vi "Pattern  Gen Test.vi"() -> ()   [LabVIEW 2016]
uses:
  Classes/Config_Read/Config_Read.lvclass
  Classes/BML_Frame_SetID/BML_Frame_SetID.lvclass
  C:/Users/Zijun/Desktop/zijun_PXI_dev/Solutions/5g_eap/trunk/1.0/HiSi5GmmWave/BML_Pattern_Gen_Refactor/Classes/BML_Frame_Root/BML_Frame_Root.lvclass
  Classes/Config_Read/Frame_Data.ctl
  Classes/Config_Read/OperationMode.ctl
  Classes/Config_Read/BurstLength.ctl
  Classes/Config_Read/RW_Option.ctl
  Classes/BML_DigiPattern_Generator/BML_DigiPattern_Generator.lvclass
  Classes/BML_Frame_Write/BML_Frame_Write.lvclass
  Classes/BML_Frame_RW/BML_Frame_RW.lvclass
panel:
  out "error out":errorcluster
  in  "PinMap":path
  in  "ChipID":u8
  in  "Config Path":path
  in  "error in (no error)":errorcluster
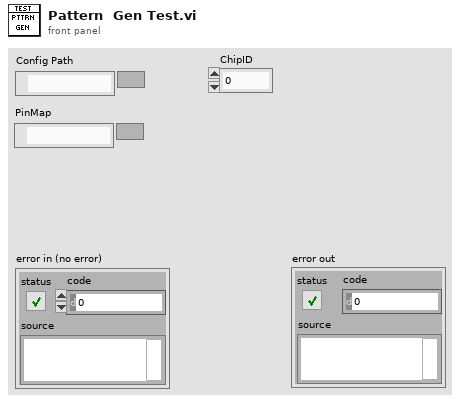
[diagram p1: front panel]
types:
  T1 = typedef "Config_Read.lvclass/Frame_Data.ctl" = cluster{"Pattern_Name":string, "Operation Mode":T2, "BurstLength":T3, "FSN":u8, "Start_Addr":u16, "Data":u8[], "R/W?":T4}
  T2 = typedef "Config_Read.lvclass/OperationMode.ctl" = enum8{"Normal", "ImmeEffect", "InitSlaveID", "LoadData"}
  T3 = typedef "Config_Read.lvclass/BurstLength.ctl" = enum8{"0", "2", "3", "4", "5", "8", "16", "32"}
  T4 = typedef "Config_Read.lvclass/RW_Option.ctl" = enum16{"Read", "Write", "R/W"}
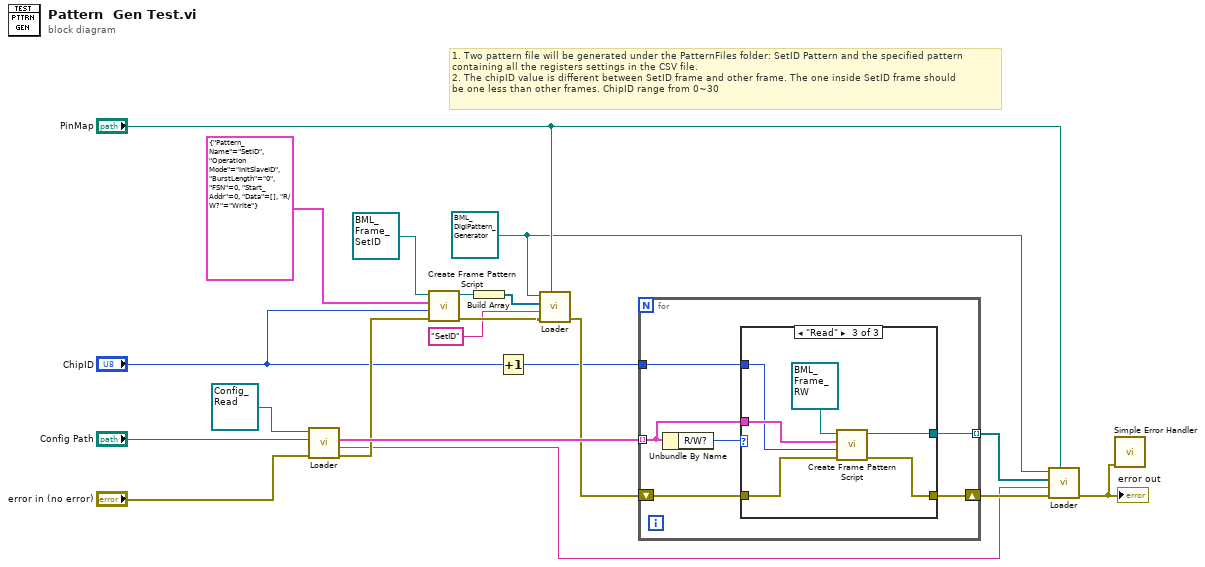
[diagram p0: block diagram]
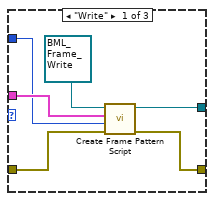
[diagram p2: hidden frame]
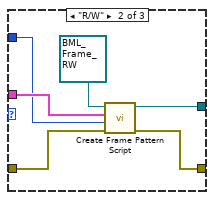
[diagram p3: hidden frame]
diagram:
  w2 = refnum<class "BML_DigiPattern_Generator.lvclass"> refnum ("BML_DigiPattern_Generator.lvclass")
  # "1. Two pattern file will be generated under the PatternFiles folder: SetID Pattern and the specified pattern\ncontaining all the registers settings in the CSV file.\n2. The chipID value is different between SetID frame and other frame. The one inside SetID frame should \nbe one less than other frames. ChipID range from 0~30"
  n1 = call "Loader.vi"("error in (no error)"="error in (no error)", "Path"="Config Path", "Config_Read.lvclass"=refnum<class "Config_Read.lvclass"> refnum) -> ("error out"=w14:errorcluster, "Pattern_Name"=w3:string, "FRM_Data_Array"=w16:T1[])  [unwired: 5 in, 1 out]
  n2 = call-dynamic "Create Frame Pattern Script.vi"("error in (no error)"=w14, "ChipID"="ChipID", "Frame_Data"=T1 {"Pattern_Name"="SetID", "Operation Mode"=enum."InitSlaveID", "BurstLength"=enum."0", "FSN"=0, "Start_Addr"=0, "Data"=[], "R/W?"=enum."Write"}, "BML_Frame_SetID in"=refnum<class "BML_Frame_SetID.lvclass"> refnum ("BML_Frame_SetID.lvclass")) -> ("error out"=w12:errorcluster, "BML_Frame_SetID out"=w8:refnum<class "BML_Frame_SetID.lvclass">)  [unwired: 6 in]
  n3 = Build Array(w8) -> (w7:refnum<class "BML_Frame_SetID.lvclass">[])
  n4 = Increment(x="ChipID") -> (x+1=w9:u8)
  n5 = call "Loader.vi"("PinMap"="PinMap", "error in (no error)"=w12, "Pattern Name"="SetID", "BML Frame Array"=w7, "BML_DigiPattern_Generator.lvclass"=w2) -> ("error out"=w13:errorcluster)  [unwired: 5 in, 1 out]
  n6 = for {
    tunnel: w16 -> [w24] mode=indexing
    tunnel: w9 -> [w23]
    shift-right: [w22] -> w6
    shift-left: w13 -> [w25]
    tunnel: [w21] -> w5 mode=indexing
    n7 = Unbundle By Name(w24) -> ("R/W?"=w26:T4)
    n8 = case shown="\"Read\"" w26 {
      tunnel: w25 -> [w30 w37 w43]
      tunnel: w24 -> [w31 w38 w44]
      tunnel: w23 -> [w29 w36 w42]
      tunnel: [w28 w35 w41] -> w21
      tunnel: [w27 w34 w40] -> w22
      frame "Write" {
        n9 = call-dynamic "Create Frame Pattern Script.vi"("error in (no error)"=w30, "ChipID"=w29, "Frame_Data"=w31, "BML_Frame_Write in"=refnum<class "BML_Frame_Write.lvclass"> refnum ("BML_Frame_Write.lvclass")) -> ("error out"=w27:errorcluster, "BML_Frame_Write out"=w28:refnum<class "BML_Frame_Write.lvclass">)  [unwired: 6 in]
      }
      frame "R/W" {
        n10 = call-dynamic "Create Frame Pattern Script.vi"("error in (no error)"=w37, "ChipID"=w36, "Frame_Data"=w38, "BML_Frame_RW in"=refnum<class "BML_Frame_RW.lvclass"> refnum ("BML_Frame_RW.lvclass")) -> ("error out"=w34:errorcluster, "BML_Frame_RW out"=w35:refnum<class "BML_Frame_RW.lvclass">)  [unwired: 6 in]
      }
      frame "Read" {
        n11 = call-dynamic "Create Frame Pattern Script.vi"("error in (no error)"=w43, "ChipID"=w42, "Frame_Data"=w44, "BML_Frame_RW in"=refnum<class "BML_Frame_RW.lvclass"> refnum ("BML_Frame_RW.lvclass")) -> ("error out"=w40:errorcluster, "BML_Frame_RW out"=w41:refnum<class "BML_Frame_RW.lvclass">)  [unwired: 6 in]
      }
    }
  }
  n12 = call "Loader.vi"("PinMap"="PinMap", "error in (no error)"=w6, "Pattern Name"=w3, "BML Frame Array"=w5, "BML_DigiPattern_Generator.lvclass"=w2) -> ("error out"=w1:errorcluster)  [unwired: 5 in, 1 out]
  "error out" <- w1
  n13 = call <vilib>:"Simple Error Handler.vi"("error in (no error)"=w1) -> ()  [unwired: 4 in, 5 out]
